vi "DHE_GetSimpleRead.vi"() -> (7 "DHE_simpleread":bool)   [LabVIEW 2016]
uses:
  private/vis/DHE_VarAction.ctl
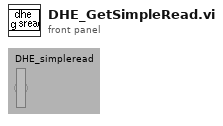
[diagram p1: front panel]
types:
  T1 = typedef "DHE_VarAction.ctl" = enum16{"read", "write"}
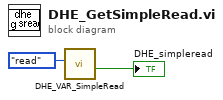
[diagram p0: block diagram]
diagram:
  n1 = call "DHE_VAR_SimpleRead.vi"("action"=DHE_VarAction."read") -> ("SimpleRead"=→"DHE_simpleread":bool)  [unwired: 1 in, 9 out]
